vi "_091.vi"() -> ()   [LabVIEW 2020]
panel:
  in  "Numeric":dbl
  # "Fundamentals"
  # "The Value in Numeric starts at 0.What is displayed in numeric after the code completes execution?"
  # "( For each run the Numeric value will be changed )"
  # "So the answer is , There is no way to tell"
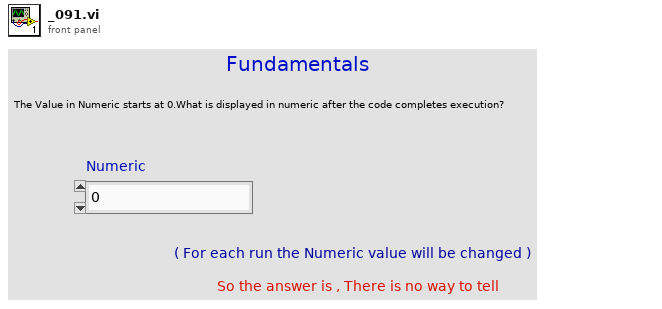
[diagram p1: front panel]
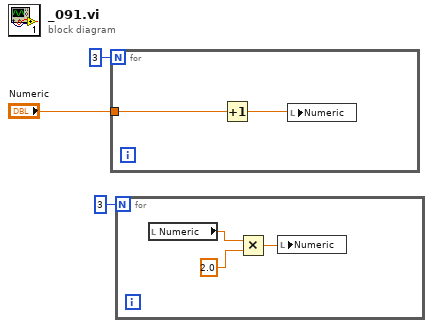
[diagram p0: block diagram]
diagram:
  n1 = for {
    N: 3 -> [_]
    tunnel: "Numeric" -> [w5]
    n2 = Increment(x=w5) -> (x+1=w4:dbl)
    n3 = local write "Numeric"(w4) -> ()
  }
  n4 = for {
    N: 3 -> [_]
    n5 = local read "Numeric"() -> (w8:dbl)
    n6 = Multiply(x=w8, y=2.0) -> (x*y=w6:dbl)
    n7 = local write "Numeric"(w6) -> ()
  }
